vi "WPI_AnalogChannelValueToVoltage.vi"(6 "Relative":bool, 8 "error in (no error)":errorcluster, 9 "Averaged":bool, 10 "Value":i32, 11 "AIDeviceRef":T1={"DevStatus"={"status"=FALSE, "code"=0, "source"=""}, "Analog Channel"=enum."AI 1"}) -> (0 "error out":errorcluster, 2 "Voltage":dbl, 3 "AIDeviceRef":T1={"DevStatus"={"status"=FALSE, "code"=0, "source"=""}, "Analog Channel"=enum."AI 1"})   [LabVIEW 2017]
uses:
  <vilib>/Rock Robotics/WPI/AnalogChannel/WPI_AnalogChannelDevRef.ctl
  <vilib>/Rock Robotics/SystemInterfaces/AI/FPGA_AIChannel.ctl
  <vilib>/Rock Robotics/SystemInterfaces/System/FPGA_SystemGet.vi
  <vilib>/Rock Robotics/SystemInterfaces/AI/FPGA_AIOversampleBits.vi
  <vilib>/Rock Robotics/SystemInterfaces/AI/FPGA_AIERRInvalidAnalogChannel.vi
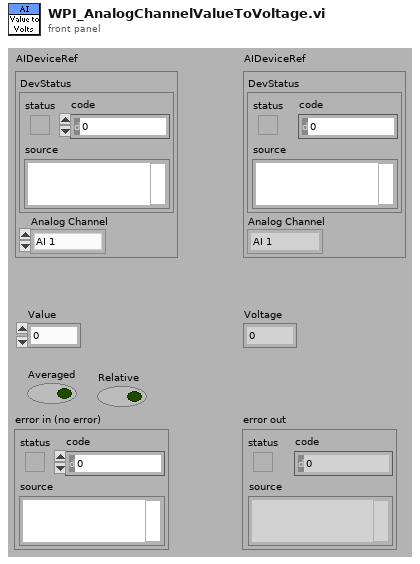
[diagram p1: front panel]
types:
  T1 = typedef "WPI_AnalogChannelDevRef.ctl" = cluster{"DevStatus":errorcluster, "Analog Channel":T2}
  T2 = typedef "FPGA_AIChannel.ctl" = enum8{"AI 0", "AI 1", "AI 2", "AI 3", "AI MXP 0", "AI MXP 1", "AI MXP 2", "AI MXP 3", "Invalid"}
  T3 = typedef "FPGA_AIDevRef.ctl" = cluster{"DevStatus":errorcluster}
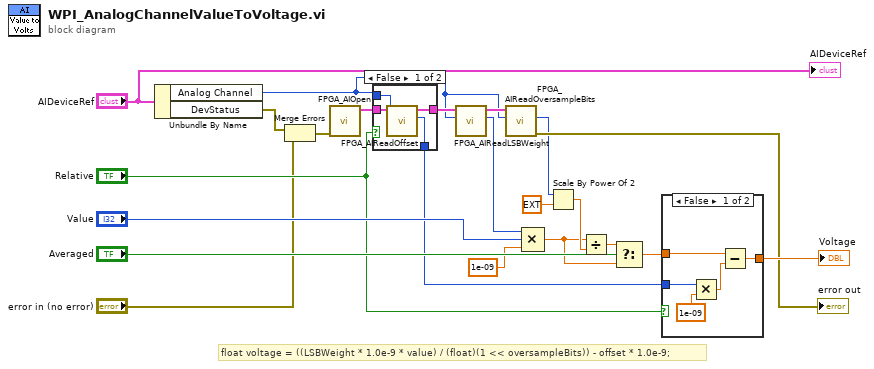
[diagram p0: block diagram]
diagram:
  # "float voltage = ((LSBWeight * 1.0e-9 * value) / (float)(1 << oversampleBits)) - offset * 1.0e-9;"
  n1 = Unbundle By Name("AIDeviceRef") -> ("Analog Channel"=w5:T2, "DevStatus"=w4:errorcluster)
  n2 = Merge Errors(w4, "error in (no error)") -> (w3:errorcluster)
  n3 = call <vilib>:"FPGA_AIOpen.vi"("error in (no error)"=w3) -> ("AI Reference out"=w13:T3)  [unwired: 2 in, 8 out]
  n4 = case shown="False" "Relative" {
    tunnel: w5 -> [w26 _]
    tunnel: [w25 w27] -> w14
    tunnel: w13 -> [w24 w27]
    tunnel: [w23 _] -> w9
    frame False {
      n5 = call <vilib>:"FPGA_AIReadOffset.vi"("Channel"=w26, "AI Reference"=w24) -> ("Offset"=w23:i32, "AI Reference"=w25:T3)  [unwired: 1 in, 7 out]
    }
    frame True {
    }
  }
  n6 = call <vilib>:"FPGA_AIReadLSBWeight.vi"("Channel"=w5, "AI Reference"=w14) -> ("LSBWeight"=w11:u32, "AI Reference"=w15:T3)  [unwired: 1 in, 7 out]
  n7 = call <vilib>:"FPGA_AIReadOversampleBits.vi"("Channel"=w5, "AI Reference in"=w15) -> ("error out"=→"error out":errorcluster, "OversampleBits"=w16:u8)  [unwired: 2 in, 6 out]
  n8 = Compound Arithmetic op=MULTIPLY(w11, "Value", 1e-09 ("y")) -> (w8:dbl)
  n9 = Scale By Power Of 2(n=w16, x=ext 1.0) -> (x*2^n=w10:ext)
  n10 = Divide(x=w8, y=w10) -> (x/y=w7:ext)
  n11 = Select(t=w7, s="Averaged", f=w8) -> (s? t:f=w6:ext)
  n12 = case shown="False" "Relative" {
    tunnel: w9 -> [w31 _]
    tunnel: w6 -> [w30 w33]
    tunnel: [w29 w33] -> w21
    frame False {
      n13 = Multiply(x=w31, y=1e-09) -> (x*y=w32:dbl)
      n14 = Subtract(x=w30, y=w32) -> (x-y=w29:ext)
    }
    frame True {
    }
  }
  "Voltage" <- w21
  "AIDeviceRef" <- "AIDeviceRef"
